vi "Render.vi"(8 "error in (no error)":errorcluster, 10 "String in":string, 11 "Heading in":refnum<class "Heading.lvclass">) -> (0 "error out":errorcluster, 2 "String out":string, 3 "Heading out":refnum<class "Heading.lvclass">)   [LabVIEW 2021, in "LvMarkdown.lvlib" / "Heading.lvclass"]
uses:
  Heading.lvclass
  C:/GitHub/LvMarkdown/src/LvMarkdown/Markdown.lvclass
  Heading.lvclass/Heading.ctl
  GetHeadingLevel.vi
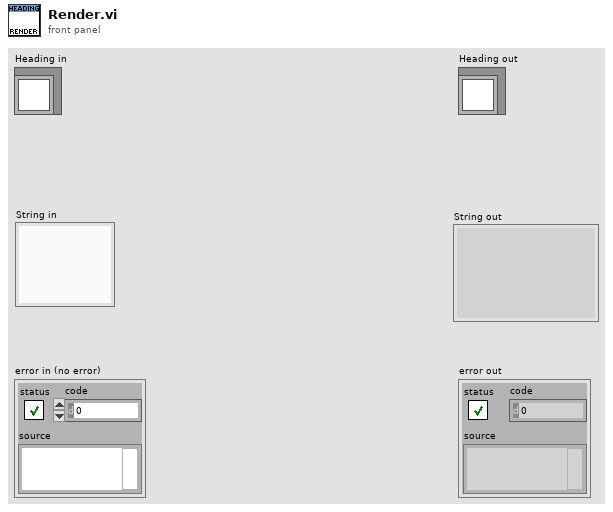
[diagram p1: front panel]
types:
  T1 = enum16{"Level 1", "Level 2", "Level 3", "Level 4", "Level 5", "Level 6"}
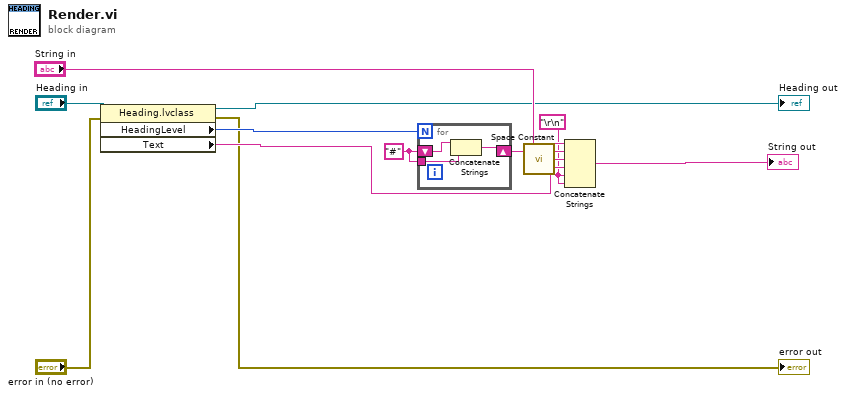
[diagram p0: block diagram]
diagram:
  w3 = "\r\n"
  w10 = "#"
  n1 = property class="Heading.lvclass"(reference="Heading in", error in="error in (no error)") -> (reference out=→"Heading out":refnum<class "Heading.lvclass">, error out=→"error out":errorcluster, "HeadingLevel"=w7:T1, "Text"=w6:string)
  n2 = for {
    N: w7 -> [_]
    shift-right: [w15] -> w9
    shift-left: w10 -> [w14]
    tunnel: w10 -> [w13]
    n3 = Concatenate Strings(w14, w13) -> (w15:string)
  }
  n4 = call <vilib>:"Space Constant.vi"() -> ("String"=w8:string)
  n5 = Concatenate Strings("String in", w9, w8, w6, w3, w3) -> (→"String out":string)
